vi "p1.vi"() -> ()   [LabVIEW 2023, in "d18.lvlib"]
uses:
  d18.lvlib
  AOC/AOC.lvlib
  <vilib>/Analysis/NI_AAL_Geometry.lvlib
panel:
  out "XY Graph":cluster{dbl[], dbl[]}[](graph)
  in  "Example":string="R 6 (#70c710)\nD 5 (#0dc571)\nL 2 (#5713f0)\nD 2 (#d2c081)\nR 2 (#59c680)\nD 2 (#411b91)\nL 5 (#8ceee2)\nU 2 (#caa173)\nL 1 (#1b58a2)\nU 2 (#caa171)\nR 2 (#7807d2)\nU 3 (#a77fa3)\nL 2 (#015232)\nU 2 (#7a21e3)"
  in  "Example":bool
  out "Answer":u64
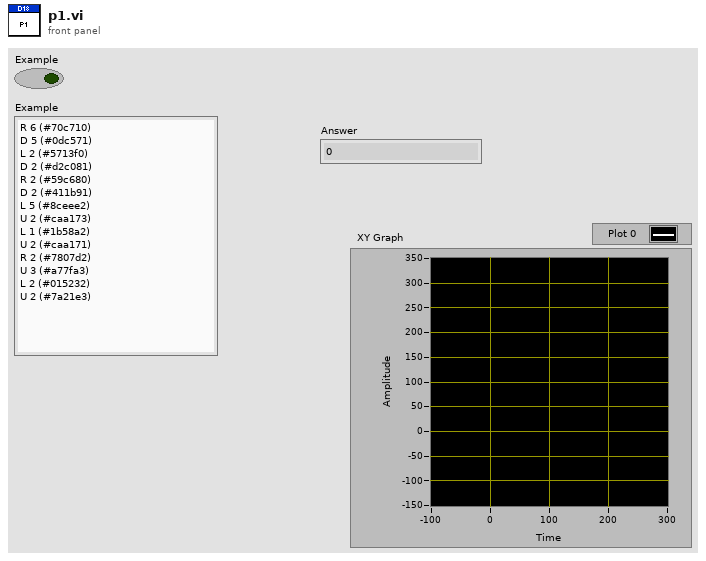
[diagram p1: front panel]
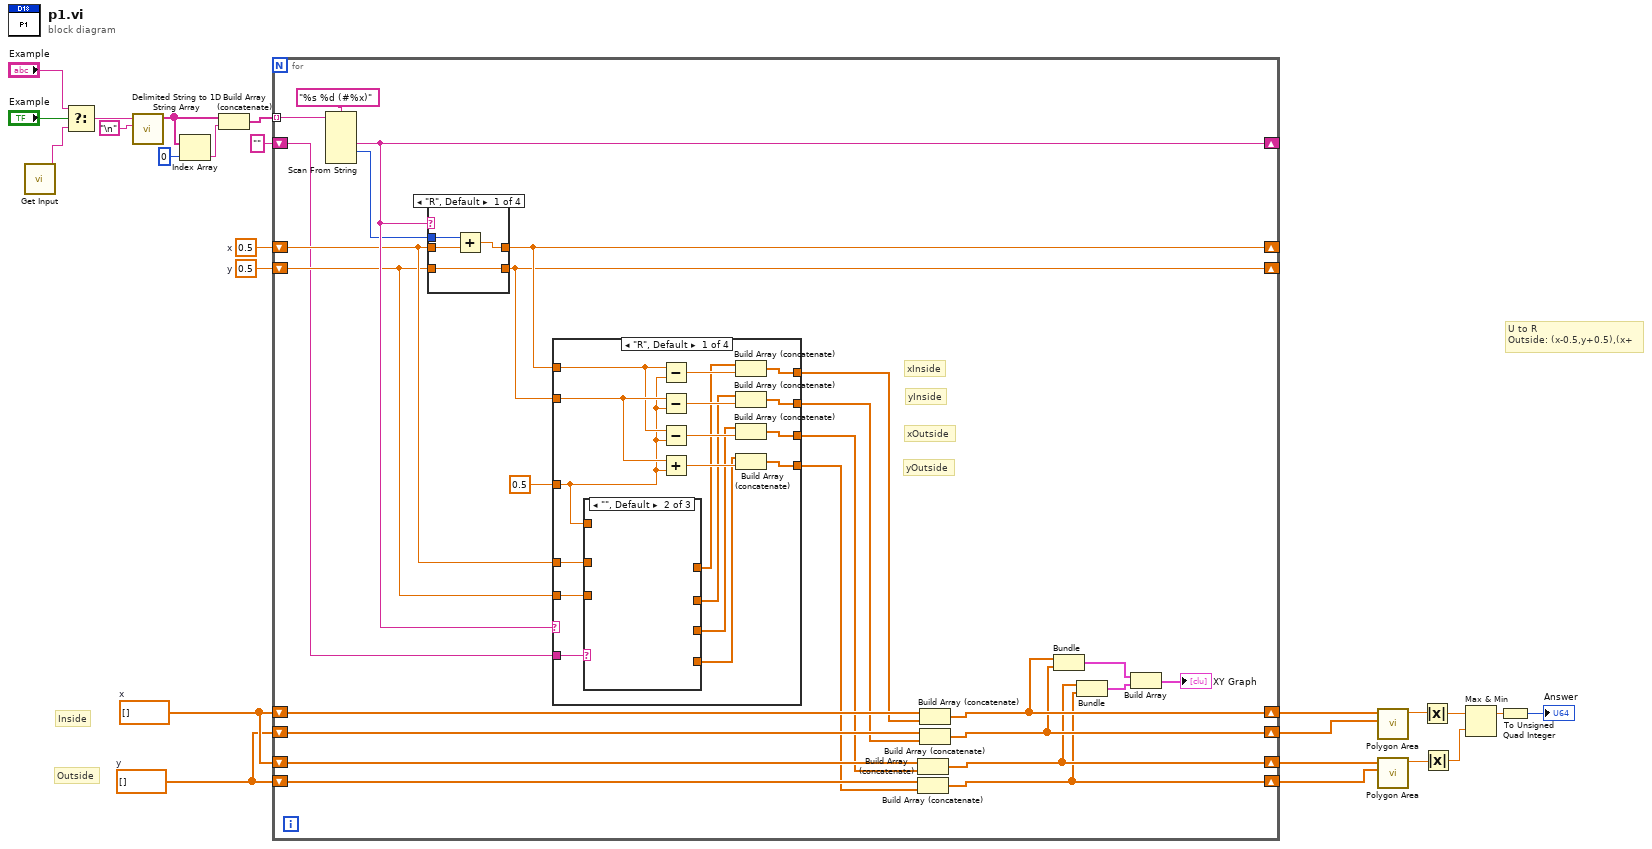
[diagram p0: block diagram]
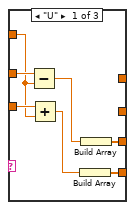
[diagram p2: hidden frame]
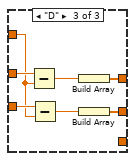
[diagram p3: hidden frame]
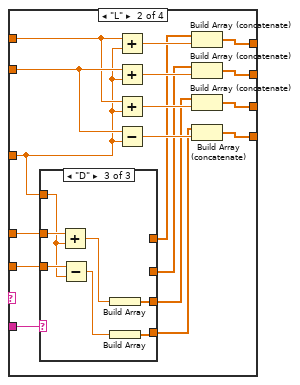
[diagram p4: hidden frame]
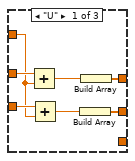
[diagram p5: hidden frame]
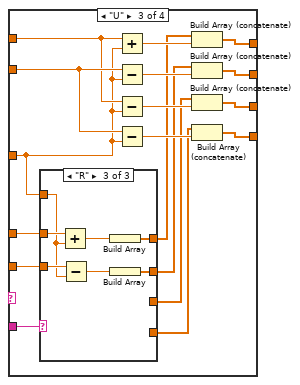
[diagram p7: hidden frame]
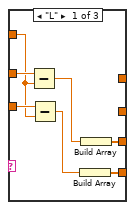
[diagram p8: hidden frame]
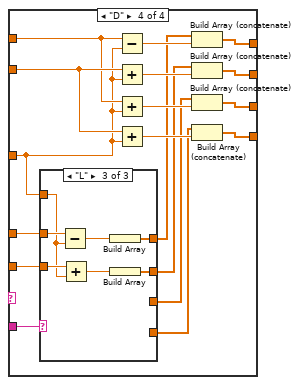
[diagram p10: hidden frame]
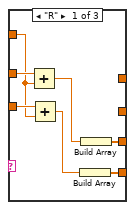
[diagram p11: hidden frame]
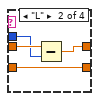
[diagram p13: hidden frame]
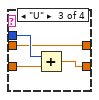
[diagram p14: hidden frame]
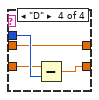
[diagram p15: hidden frame]
diagram:
  w18 = 0.5  # y
  w19 = 0.5  # x
  w14 = dbl[] []  # y
  w15 = dbl[] []  # x
  # "Outside"
  # "Inside"
  # "U to R\nOutside: (x-0.5,y+0.5),(x+"
  n1 = call "Get Input.vi"() -> ("Input"=w24:string)  [unwired: 11 in]
  n2 = Select(t="Example", s="Example", f=w24) -> (s? t:f=w23:string)
  n3 = call <vilib>:"Delimited String to 1D String Array.vi"("delimiter"="\n", "delimited string"=w23) -> ("string array"=w4:string[])  [unwired: 9 in]
  n4 = Index Array(array=w4, index=0) -> (element=w1:string)
  n5 = Build Array (concatenate)(w4, w1) -> (w2:string[])
  n6 = for {
    tunnel: w2 -> [w49] mode=indexing
    shift-right: [w31] -> w6
    shift-left: w15 -> [w47]
    shift-right: [w30] -> w5
    shift-left: w14 -> [w46]
    shift-right: [w40] -> _
    shift-left: w18 -> [w33]
    shift-right: [w42] -> _
    shift-left: w19 -> [w34]
    shift-right: [w29] -> w12
    shift-left: w15 -> [w45]
    shift-right: [w28] -> w11
    shift-left: w14 -> [w44]
    shift-right: [w43] -> _
    shift-left: "" -> [w32]
    # "yOutside"
    # "yInside"
    # "xOutside"
    # "xInside"
    n7 = Scan From String(format string="%s %d (#%x)", input string=w49) -> (output 1=w43:string, output 2=w41:i32)  [unwired: 6 in, 3 out]
    n8 = case shown="\"R\", Default" w43 {
      tunnel: w34 -> [w181 w185 w186 w190]
      tunnel: w33 -> [w178 w182 w188 w192]
      tunnel: w41 -> [w180 w184 w189 w193]
      tunnel: [w179 w183 w186 w190] -> w42
      tunnel: [w178 w182 w187 w191] -> w40
      frame "R", Default {
        n9 = Add(x=w180, y=w181) -> (x+y=w179:dbl)
      }
      frame "L" {
        n10 = Subtract(x=w185, y=w184) -> (x-y=w183:dbl)
      }
      frame "U" {
        n11 = Add(x=w189, y=w188) -> (x+y=w187:dbl)
      }
      frame "D" {
        n12 = Subtract(x=w192, y=w193) -> (x-y=w191:dbl)
      }
    }
    n13 = case shown="\"R\", Default" w43 {
      tunnel: w42 -> [w60 w91 w123 w155]
      tunnel: [w67 w99 w131 w163] -> w39
      tunnel: [w66 w98 w129 w161] -> w38
      tunnel: [w65 w97 w128 w160] -> w37
      tunnel: [w64 w96 w127 w159] -> w36
      tunnel: w40 -> [w62 w94 w125 w157]
      tunnel: 0.5 ("y") -> [w54 w87 w118 w150]
      tunnel: w34 -> [w56 w90 w119 w151]
      tunnel: w33 -> [w55 w89 w120 w152]
      tunnel: w32 -> [w57 w88 w121 w153]
      frame "R", Default {
        n14 = case shown="\"\", Default" w57 {
          tunnel: w56 -> [w74 _ w81]
          tunnel: w55 -> [w73 _ w80]
          tunnel: w54 -> [w72 _ w79]
          tunnel: [_ _ w77] -> w53
          tunnel: [_ _ w75] -> w52
          tunnel: [w68 _ _] -> w51
          tunnel: [w69 _ _] -> w50
          frame "U" {
            n15 = Subtract(x=w74, y=w72) -> (x-y=w71:dbl)
            n16 = Add(x=w73, y=w72) -> (x+y=w70:dbl)
            n17 = Build Array(w70) -> (w69:dbl[])
            n18 = Build Array(w71) -> (w68:dbl[])
          }
          frame "", Default {
          }
          frame "D" {
            n19 = Subtract(x=w81, y=w79) -> (x-y=w78:dbl)
            n20 = Subtract(x=w80, y=w79) -> (x-y=w76:dbl)
            n21 = Build Array(w78) -> (w77:dbl[])
            n22 = Build Array(w76) -> (w75:dbl[])
          }
        }
        n23 = Subtract(x=w60, y=w54) -> (x-y=w58:dbl)
        n24 = Subtract(x=w62, y=w54) -> (x-y=w63:dbl)
        n25 = Subtract(x=w60, y=w54) -> (x-y=w59:dbl)
        n26 = Add(x=w62, y=w54) -> (x+y=w61:dbl)
        n27 = Build Array (concatenate)(w53, w58) -> (w67:dbl[])
        n28 = Build Array (concatenate)(w52, w63) -> (w65:dbl[])
        n29 = Build Array (concatenate)(w51, w59) -> (w66:dbl[])
        n30 = Build Array (concatenate)(w50, w61) -> (w64:dbl[])
      }
      frame "L" {
        n31 = case shown="\"D\"" w88 {
          tunnel: w90 -> [w106 _ w113]
          tunnel: w89 -> [w105 _ w112]
          tunnel: w87 -> [w104 _ w111]
          tunnel: [w100 _ _] -> w85
          tunnel: [w101 _ _] -> w84
          tunnel: [_ _ w108] -> w83
          tunnel: [_ _ w107] -> w82
          frame "U" {
            n32 = Add(x=w106, y=w104) -> (x+y=w103:dbl)
            n33 = Add(x=w105, y=w104) -> (x+y=w102:dbl)
            n34 = Build Array(w102) -> (w101:dbl[])
            n35 = Build Array(w103) -> (w100:dbl[])
          }
          frame "", Default {
          }
          frame "D" {
            n36 = Add(x=w113, y=w111) -> (x+y=w110:dbl)
            n37 = Subtract(x=w112, y=w111) -> (x-y=w109:dbl)
            n38 = Build Array(w110) -> (w108:dbl[])
            n39 = Build Array(w109) -> (w107:dbl[])
          }
        }
        n40 = Add(x=w91, y=w87) -> (x+y=w86:dbl)
        n41 = Add(x=w94, y=w87) -> (x+y=w95:dbl)
        n42 = Add(x=w91, y=w87) -> (x+y=w92:dbl)
        n43 = Subtract(x=w94, y=w87) -> (x-y=w93:dbl)
        n44 = Build Array (concatenate)(w85, w86) -> (w99:dbl[])
        n45 = Build Array (concatenate)(w84, w95) -> (w97:dbl[])
        n46 = Build Array (concatenate)(w83, w92) -> (w98:dbl[])
        n47 = Build Array (concatenate)(w82, w93) -> (w96:dbl[])
      }
      frame "U" {
        n48 = case shown="\"R\"" w121 {
          tunnel: w119 -> [w138 _ w145]
          tunnel: w120 -> [w137 _ w144]
          tunnel: w118 -> [w136 _ w143]
          tunnel: [_ _ w141] -> w117
          tunnel: [_ _ w139] -> w116
          tunnel: [w132 _ _] -> w115
          tunnel: [w133 _ _] -> w114
          frame "L" {
            n49 = Subtract(x=w138, y=w136) -> (x-y=w135:dbl)
            n50 = Subtract(x=w137, y=w136) -> (x-y=w134:dbl)
            n51 = Build Array(w134) -> (w133:dbl[])
            n52 = Build Array(w135) -> (w132:dbl[])
          }
          frame "", Default {
          }
          frame "R" {
            n53 = Add(x=w145, y=w143) -> (x+y=w142:dbl)
            n54 = Subtract(x=w144, y=w143) -> (x-y=w140:dbl)
            n55 = Build Array(w142) -> (w141:dbl[])
            n56 = Build Array(w140) -> (w139:dbl[])
          }
        }
        n57 = Add(x=w123, y=w118) -> (x+y=w130:dbl)
        n58 = Subtract(x=w125, y=w118) -> (x-y=w126:dbl)
        n59 = Subtract(x=w123, y=w118) -> (x-y=w122:dbl)
        n60 = Subtract(x=w125, y=w118) -> (x-y=w124:dbl)
        n61 = Build Array (concatenate)(w117, w130) -> (w131:dbl[])
        n62 = Build Array (concatenate)(w116, w126) -> (w128:dbl[])
        n63 = Build Array (concatenate)(w115, w122) -> (w129:dbl[])
        n64 = Build Array (concatenate)(w114, w124) -> (w127:dbl[])
      }
      frame "D" {
        n65 = case shown="\"L\"" w153 {
          tunnel: w151 -> [w170 _ w177]
          tunnel: w152 -> [w169 _ w176]
          tunnel: w150 -> [w168 _ w175]
          tunnel: [_ _ w173] -> w149
          tunnel: [_ _ w171] -> w148
          tunnel: [w164 _ _] -> w147
          tunnel: [w165 _ _] -> w146
          frame "R" {
            n66 = Add(x=w170, y=w168) -> (x+y=w167:dbl)
            n67 = Add(x=w169, y=w168) -> (x+y=w166:dbl)
            n68 = Build Array(w166) -> (w165:dbl[])
            n69 = Build Array(w167) -> (w164:dbl[])
          }
          frame "", Default {
          }
          frame "L" {
            n70 = Subtract(x=w177, y=w175) -> (x-y=w174:dbl)
            n71 = Add(x=w176, y=w175) -> (x+y=w172:dbl)
            n72 = Build Array(w174) -> (w173:dbl[])
            n73 = Build Array(w172) -> (w171:dbl[])
          }
        }
        n74 = Subtract(x=w155, y=w150) -> (x-y=w162:dbl)
        n75 = Add(x=w157, y=w150) -> (x+y=w158:dbl)
        n76 = Add(x=w155, y=w150) -> (x+y=w154:dbl)
        n77 = Add(x=w157, y=w150) -> (x+y=w156:dbl)
        n78 = Build Array (concatenate)(w149, w162) -> (w163:dbl[])
        n79 = Build Array (concatenate)(w148, w158) -> (w160:dbl[])
        n80 = Build Array (concatenate)(w147, w154) -> (w161:dbl[])
        n81 = Build Array (concatenate)(w146, w156) -> (w159:dbl[])
      }
    }
    n82 = Build Array (concatenate)(w45, w38) -> (w29:dbl[])
    n83 = Build Array (concatenate)(w44, w36) -> (w28:dbl[])
    n84 = Build Array (concatenate)(w47, w39) -> (w31:dbl[])
    n85 = Build Array (concatenate)(w46, w37) -> (w30:dbl[])
    n86 = Bundle(w31, w30) -> (w27:cluster{dbl[], dbl[]})  [unwired: 1 in]
    n87 = Bundle(w29, w28) -> (w26:cluster{dbl[], dbl[]})  [unwired: 1 in]
    n88 = Build Array(w27, w26) -> (→"XY Graph":cluster{dbl[], dbl[]}[])
  }
  n89 = call <vilib>:"Polygon Area.vi"("Y"=w5, "X"=w6) -> ("signed area"=w17:dbl)  [unwired: 8 in, 1 out]
  n90 = call <vilib>:"Polygon Area.vi"("Y"=w11, "X"=w12) -> ("signed area"=w10:dbl)  [unwired: 8 in, 1 out]
  n91 = Absolute Value(x=w17) -> (abs(x)=w8:dbl)
  n92 = Absolute Value(x=w10) -> (abs(x)=w9:dbl)
  n93 = Max & Min(x=w8, y=w9) -> (max(x,y)=w7:dbl)  [unwired: 1 out]
  n94 = To Unsigned Quad Integer(1:w7) -> (0:→"Answer":u64)
